vi "On New Window Requested.vi"(8 "error in (no error)":errorcluster, 10 "Data":T1, 11 "WebView2 Event Filter Interface in":refnum<class "WebView2 Event Filter Interface.lvclass">) -> (0 "error out":errorcluster, 1 "NewWindow":refnum<k24>, 2 "Handled":bool)   [LabVIEW 2025, in "WebView2.lvlib" / "WebView2 Event Filter Interface.lvclass"]
uses:
  WebView2 Event Filter Interface.lvclass
  WebView2 Control Object/New Window Event Data.ctl
  E:/Labview/LV 2023/PPL/PPL Builder/Libs/LV-WebView2/Source/Libs/Microsoft.Web.WebView2.Core.dll
  Libs/Microsoft.Web.WebView2.Core.dll
  WebView2 Control Object/WebView2 Control.lvclass
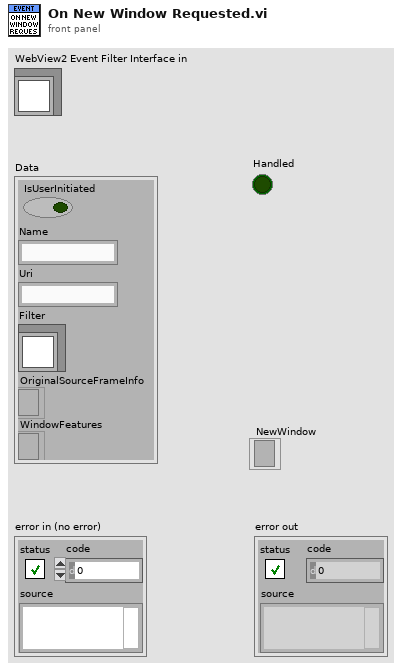
[diagram p1: front panel]
types:
  T1 = typedef "WebView2.lvlib/WebView2 Control.lvclass/New Window Event Data.ctl" = cluster{"IsUserInitiated":bool, "Name":string, "Uri":string, "Filter":refnum<class "WebView2 Event Filter Interface.lvclass">, "OriginalSourceFrameInfo":refnum<k24>, "WindowFeatures":refnum<k24>}
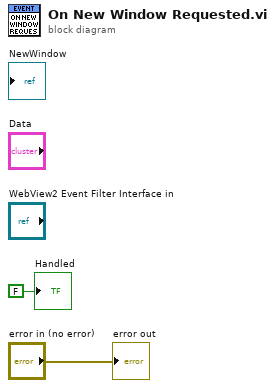
[diagram p0: block diagram]
diagram:
  "error out" <- "error in (no error)"
  "Handled" <- FALSE ("Handled")
